vi "Executable Auto Increment Build Version__icon_lib_labview_project_api.vi"(8 "error in (no error)":errorcluster, 11 "Build Spec Reference":refnum<vi>) -> (0 "error out":errorcluster, 3 "Build Spec Reference Dup":refnum<vi>)   [LabVIEW 2016, in "LabVIEW Project API__icon_lib_labview_project_api.lvlib"]
doc: "Increments the Build Specification Executable Version [Major, Minor, Fix, Build] by 1. Major, Minor and Fix are unchanged.\n\n<b>Author:</b> JG\n\n<b>ICON Technologies Pty Ltd</b>\nCopyright (C) 1990-2009\nAll Rights Reserved"
uses:
  LabVIEW Project API__icon_lib_labview_project_api.lvlib
panel:
  # "Output"
  # "Input"
  # "ICON Technologies Pty Ltd\nCopyright (C) 1990-2009\nAll Rights Reserved"
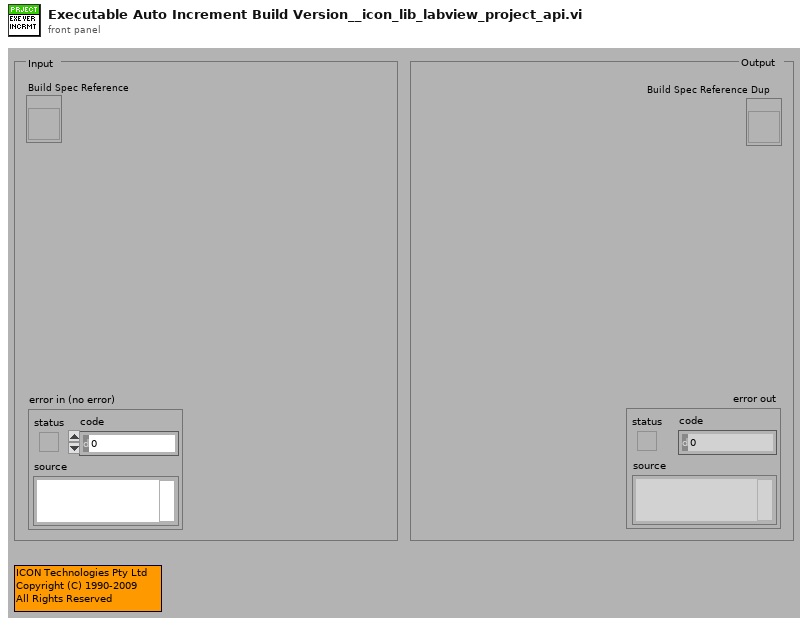
[diagram p1: front panel]
types:
  T1 = cluster{"Major":u16, "Minor":u16, "Fix":u16, "Build":u16}
  T2 = cluster{"Version[0]":u16, "Version[1]":u16, "Version[2]":u16, "Version[3]":u16}
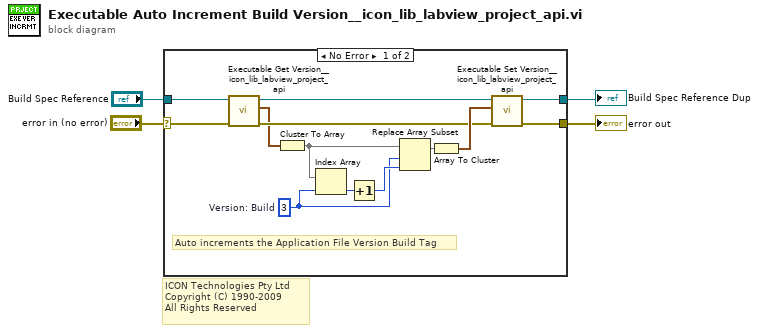
[diagram p0: block diagram]
diagram:
  # "ICON Technologies Pty Ltd\nCopyright (C) 1990-2009\nAll Rights Reserved"
  n1 = case shown="No Error" "error in (no error)" {
    selector: "error in (no error)" -> [w7 w19]
    tunnel: [w6 w19] -> w3
    tunnel: "Build Spec Reference" -> [w8 w18]
    tunnel: [w5 w18] -> w1
    frame No Error {
      w15 = 3  # Version: Build
      # "Auto increments the Application File Version Build Tag"
      n2 = call "Executable Get Version__icon_lib_labview_project_api.vi"("error in (no error)"=w7, "Build Spec Reference"=w8) -> ("error out"=w13:errorcluster, "Version"=w9:T1, "Build Spec Reference Dup"=w14:refnum<vi>)  [unwired: 7 out]
      n3 = Cluster To Array(cluster=w9) -> (array=w11:u16[])
      n4 = Index Array(array=w11, index=w15) -> (element=w10:u16)
      n5 = Increment(x=w10) -> (x+1=w17:u16)
      n6 = Replace Array Subset(array=w11, new element=w17, index=w15) -> (w12:u16[])
      n7 = Array To Cluster(array=w12) -> (cluster=w16:T2)
      n8 = call "Executable Set Version__icon_lib_labview_project_api.vi"("error in (no error)"=w13, "Version"=w16, "Build Spec Reference"=w14) -> ("error out"=w6:errorcluster, "Build Spec Reference Dup"=w5:refnum<vi>)  [unwired: 7 out]
    }
    frame Error {
    }
  }
  "error out" <- w3
  "Build Spec Reference Dup" <- w1
